vi "Configure Trigger.vi"(8 "error in (no error)":errorcluster, 10 "Trigger Value (00000)":i16 format="%05.0f", 11 "VISA resource name":refnum<visa-resource-name>) -> (0 "error out":errorcluster, 3 "VISA resource name out":refnum<visa-resource-name>)   [LabVIEW 2016, in "EFD Ultimus V.lvlib"]
doc: "This VI downloads the 5-digit trigger value into the current memory location.\n\nHost Format: EQ--Tttttt\nttttt:Trigger Value 000001-99999"
uses:
  EFD Ultimus V.lvlib
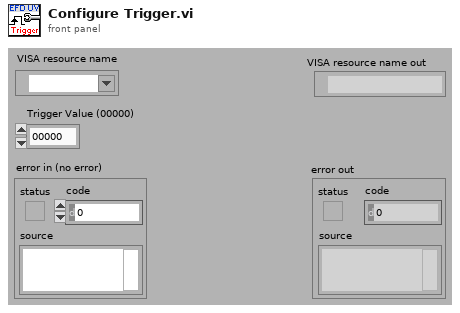
[diagram p1: front panel]
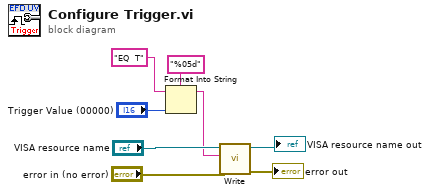
[diagram p0: block diagram]
diagram:
  n1 = Format Into String(format string="%05d", initial string="EQ  T" ("string"), "Trigger Value (00000)") -> (resulting string=w3:string)  [unwired: 1 in, 1 out]
  n2 = call "Write.vi"("error in (no error)"="error in (no error)", "Command To Write"=w3, "VISA resource name"="VISA resource name") -> ("error out"=→"error out":errorcluster, "VISA resource name out"=→"VISA resource name out":refnum<visa-resource-name>)  [unwired: 7 out]
